vi "Parser.vi"() -> ()   [LabVIEW 2015]
uses:
  Components/YAML Parser Class/YAML Parser.lvclass
panel:
  in  "YAML Tree":string(tree)
  out "error out":errorcluster
  in  "YAML String":string="  name:   \"Nicolas\"\n  age:                  27.500000\n  \"age en jours\":   1234\n  address:              \r\n    city:            \"Grenoble\"\n    postal-code:     \"38000\"\n    street:          \"rue Jean Prevost\"\n  commentaires:         ~"
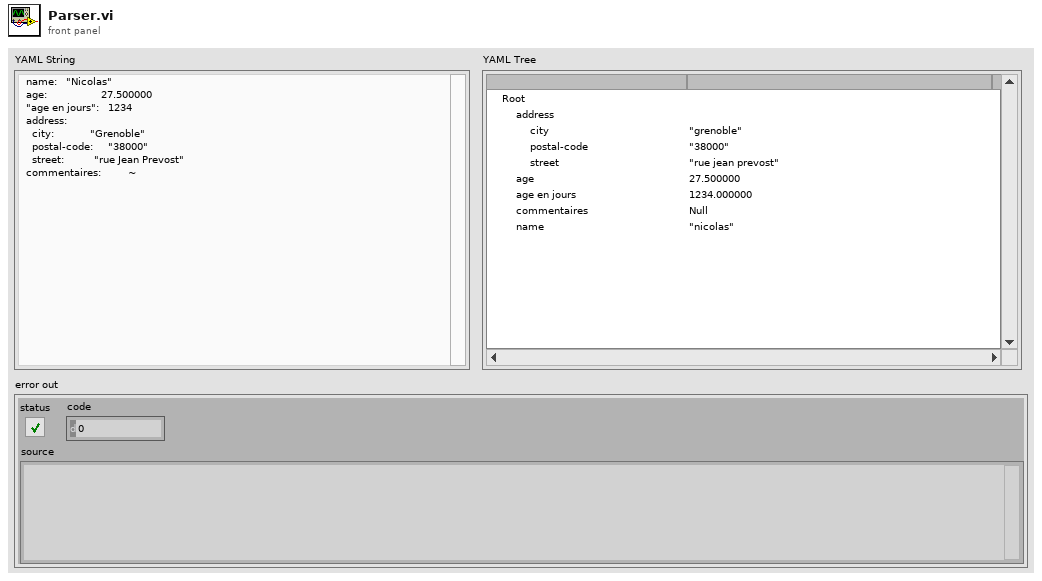
[diagram p1: front panel]
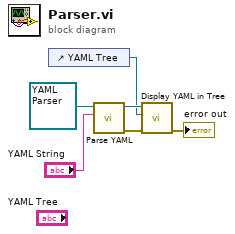
[diagram p0: block diagram]
diagram:
  n1 = control-ref of="YAML Tree"() -> (w3:refnum<vi>)
  n2 = call "Parse YAML.vi"("YAML String"="YAML String", "YAML Parser in"=refnum<class "YAML Parser.lvclass"> refnum) -> ("error out"=w2:errorcluster, "YAML Parser out"=w4:refnum<class "YAML Parser.lvclass">)  [unwired: 8 in]
  n3 = call "Display YAML in Tree.vi"("error in (no error)"=w2, "Tree Refnum"=w3, "YAML Parser in"=w4) -> ("error out"=→"error out":errorcluster)  [unwired: 7 in, 1 out]
